vi "GetBoolValue.vi"(2 "error in (no error)":errorcluster, 3 "Feature Name":string, 4 "IGxDevice":refnum<k24>) -> (0 "error out":errorcluster, 1 "Bool Value":bool)   [LabVIEW 2013, in "GxLVlib.lvlib"]
uses:
  GxLVlib.lvlib
  F:/GxILibrary/Labview/trunk/private/dev/src/C#/x86/GxLVLib/dll/GxIAPINET.dll
  private/dev/src/C#/x86/GxLVLib/dll/GxIAPINET.dll
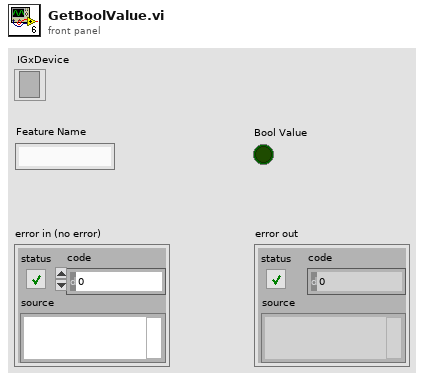
[diagram p1: front panel]
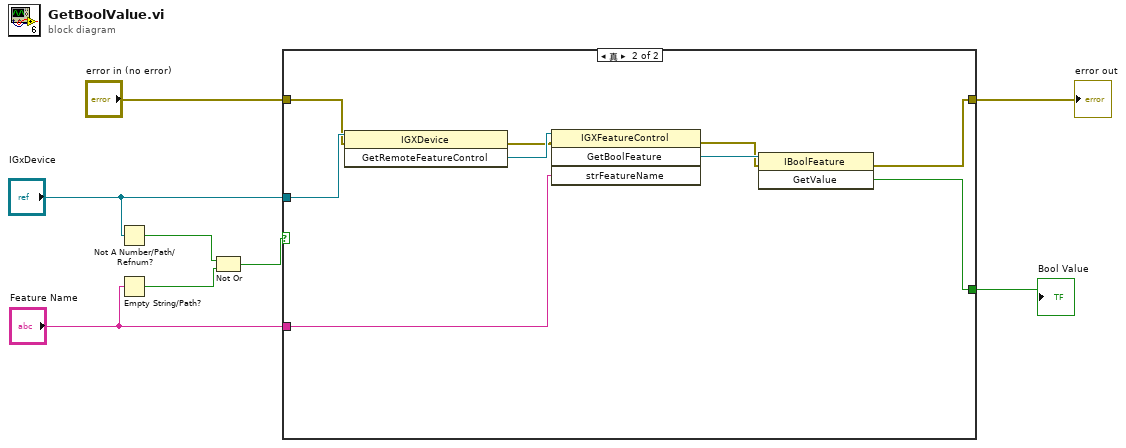
[diagram p0: block diagram]
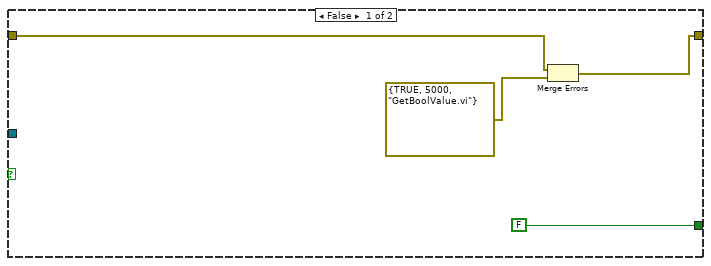
[diagram p2: hidden frame]
diagram:
  n1 = Not A Number/Path/Refnum?(number/path/refnum="IGxDevice") -> (NaN/Path/Refnum?=w8:bool)
  n2 = Empty String/Path?(string/path="Feature Name") -> (empty?=w7:bool)
  n3 = Not Or(1:w7, 2:w8) -> (0:w6:bool)
  n4 = case shown="真" w6 {
    tunnel: "error in (no error)" -> [w11 w19]
    tunnel: [w10 w13] -> w4
    tunnel: [FALSE w15] -> w3
    tunnel: "IGxDevice" -> [_ w21]
    tunnel: "Feature Name" -> [_ w17]
    frame False {
      n5 = Merge Errors(w11, errorcluster {TRUE, 5000, "GetBoolValue.vi"}) -> (w10:errorcluster)
    }
    frame True {
      n6 = invoke class="IGXDevice" method="GetRemoteFeatureControl"(reference=w21, error in=w19) -> (error out=w18:errorcluster, "GetRemoteFeatureControl"=w20:refnum<k24>)  [unwired: 1 in, 1 out]
      n7 = invoke class="IGXFeatureControl" method="GetBoolFeature"(reference=w20, error in=w18, "strFeatureName"=w17) -> (error out=w14:errorcluster, "GetBoolFeature"=w16:refnum<k24>)  [unwired: 1 in, 2 out]
      n8 = invoke class="IBoolFeature" method="GetValue"(reference=w16, error in=w14) -> (error out=w13:errorcluster, "GetValue"=w15:bool)  [unwired: 1 in, 1 out]
    }
  }
  "error out" <- w4
  "Bool Value" <- w3
